vi "Joystick Program.vi"() -> ()   [LabVIEW 2014]
uses:
  <vilib>/Rock Robotics/WPI/Joystick/WPI_JoystickDeviceEnum.ctl
  <vilib>/Utility/inputDevices.llb/joystickAcquire.vi
  <vilib>/Utility/inputDevices.llb/closeJoystick.vi
panel:
  out "Z axis rotation":i32
  out "U axis":i32
  out "HAT":i32
  out "button 12":bool
  out "button 11":bool
  out "button 10":bool
  out "button 9":bool
  out "button 8":bool
  out "Y axis":i32
  out "X axis":i32
  out "button 7":bool
  out "button 6":bool
  out "button 5":bool
  out "button 4":bool
  out "button 3":bool
  in  "stop":bool
  out "button 2":bool
  out "button 1":bool
  # "Z-Axis Rotation is the Rotation\n of the Joystick left and right \n(Note that it doesnt center at 0)"
  # "The HAT is an eight-way directional pad that\nis shown by the degree it faces:\nCenter = -1\nUp = 0 Down = 180\nLeft = 270 Right = 90\nUp-Right = 45 Up-Left = 315\nDown-Right = 135 Down-Left = 225"
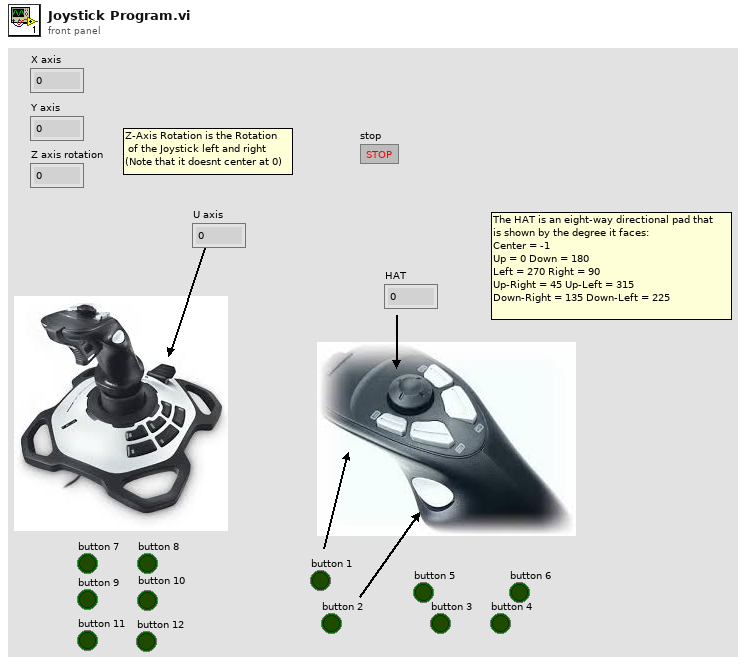
[diagram p1: front panel]
types:
  T1 = typedef "WPI_JoystickDeviceEnum.ctl" = enum16{"USB 0", "USB 1", "USB 2", "USB 3", "USB 4", "USB 5"}
  T2 = cluster{"X axis":i32, "Y axis":i32, "Z axis":i32, "X axis rotation":i32, "Y axis rotation":i32, "Z axis rotation":i32, "U axis":i32, "V axis":i32}
  T3 = cluster{"button 1":bool, "button 2":bool, "button 3":bool, "button 4":bool, "button 5":bool, "button 6":bool, "button 7":bool, "button 8":bool, "button 9":bool, "button 10":bool, "button 11":bool, "button 12":bool, "button 13":bool, "button 14":bool, "button 15":bool, "button 16":bool, "button 17":bool, "button 18":bool, "button 19":bool, "button 20":bool, "button 21":bool, "button 22":bool, "button 23":bool, "button 24":bool, "button 25":bool, "button 26":bool, "button 27":bool, "button 28":bool, "button 29":bool, "button 30":bool, "button 31":bool, "button 32":bool}
  T4 = cluster{"pov 1":i32, "pov 2":i32, "pov 3":i32, "pov 4":i32}
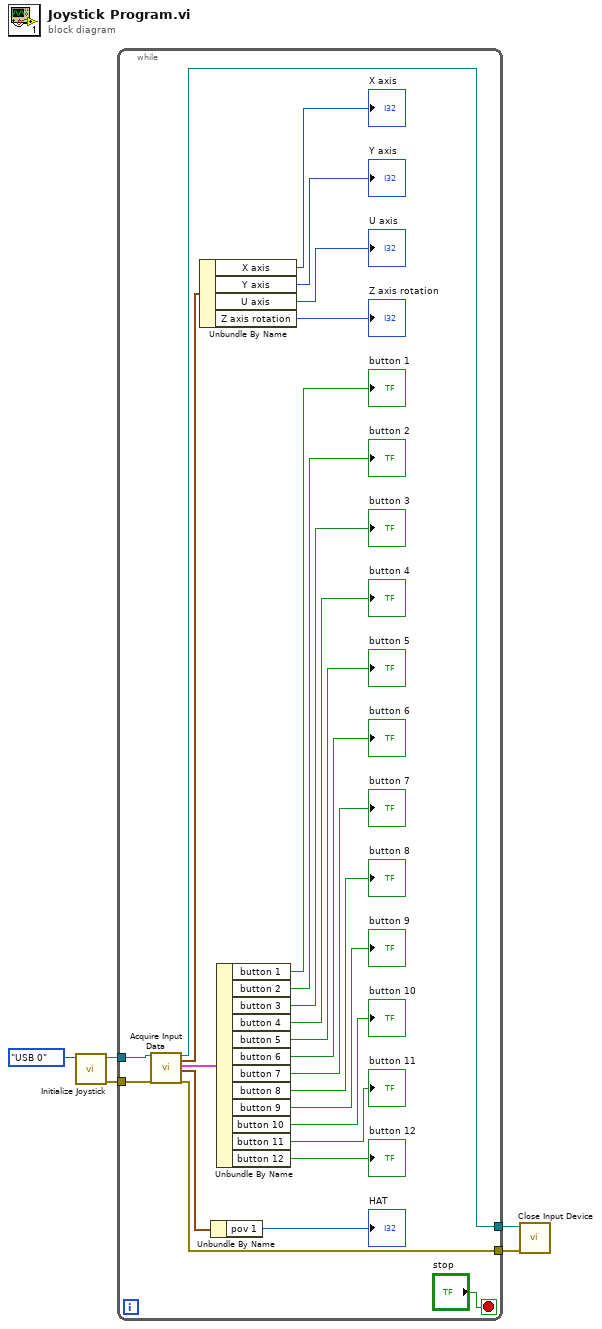
[diagram p0: block diagram]
diagram:
  n1 = call <vilib>:"Initialize Joystick.vi"("device index"=WPI_JoystickDeviceEnum."USB 0" ("JoystickDevice")) -> ("error out"=w1:errorcluster, "device ID"=w4:refnum<k1>)  [unwired: 9 in]
  n2 = while {
    tunnel: w4 -> [w17]
    tunnel: [w16] -> w3
    tunnel: [w15] -> w2
    tunnel: w1 -> [w14]
    stop <- "stop" stop-if-true
    n3 = call-poly <vilib>:"Acquire Input Data.vi"("device ID"=w17, "error in (no error)"=w14) -> ("device ID"=w16:refnum<k1>, "axis info"=w19:T2, "button info"=w18:T3, "direction info"=w8:T4, "error out"=w15:errorcluster)  [unwired: 13 in]
    n4 = Unbundle By Name(w19) -> ("X axis"=→"X axis":i32, "Y axis"=→"Y axis":i32, "U axis"=→"U axis":i32, "Z axis rotation"=→"Z axis rotation":i32)
    n5 = Unbundle By Name(w8) -> ("pov 1"=→"HAT":i32)
    n6 = Unbundle By Name(w18) -> ("button 1"=→"button 1":bool, "button 2"=→"button 2":bool, "button 3"=→"button 3":bool, "button 4"=→"button 4":bool, "button 5"=→"button 5":bool, "button 6"=→"button 6":bool, "button 7"=→"button 7":bool, "button 8"=→"button 8":bool, "button 9"=→"button 9":bool, "button 10"=→"button 10":bool, "button 11"=→"button 11":bool, "button 12"=→"button 12":bool)
  }
  n7 = call-poly <vilib>:"Close Input Device.vi"("error in (no error)"=w2, "device ID"=w3) -> ()  [unwired: 8 in, 1 out]
